vi "move_2.vi"(3 "t":bool, 4 "Array in":i32[](array[numeric]), 5 "Enum 3":enum16{"move2_1", "move2_2"}(ring)) -> (0 "Enum":T1(ring), 1 "Array out":i32[](array[numeric]), 2 "Enum 2":enum16{"move2_1", "move2_2"}(ring))   [LabVIEW 2016]
uses:
  <vilib>/NXT/Block Support/NXT_OutputPort.ctl
  <vilib>/NXT/NXTIO Xnodes/NXTIONodeSubVIs/NXTStopMotors.vi
  <vilib>/NXT/NXTIO Xnodes/NXTIONodeSubVIs/NXTMotorRunDistance.vi
  <vilib>/NXT/NXTIO Xnodes/NXTIONodeSubVIs/LEGOMotorStatus.vi
  <vilib>/NXT/NXTIO Xnodes/NXTIONodeSubVIs/NXTMoveMotors.vi
  <vilib>/NXT/NXTIO Xnodes/NXTIONodeSubVIs/LEGOResetMotors.vi
  <vilib>/NXT/Dual Mode Library/Display/drawText.vi
  <vilib>/NXT/Subs/LVHSConnector.ctl
  <vilib>/NXT/NXTIO Xnodes/AddressXNode/NXTIOAddress.xnode
  <vilib>/NXT/NXTIO Xnodes/NXTIOXNode/NXTIO.xnode
  <vilib>/NXT/LegoClasses/BrickReference/BrickReference.lvclass
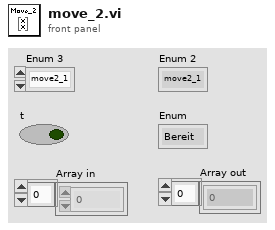
[diagram p1: front panel]
types:
  T1 = enum16{"Bereit", "Move 1", "Reference_pos", "Wait", "row1_check", "row2_check", "row3_check", "return", "move2", "move3", "move4", "move5", "end"}
  T2 = enum16{"forward", "right", "mark", "pause", "up", "return", "end"}
  T3 = typedef "NXT_OutputPort.ctl" = u8
  T4 = cluster{"Output Port":T3, "Output Port 2":T3, "Output Port 3":T3}
  T5 = enum16{"forward", "mark", "pause", "up", "return", "end"}
  T6 = typedef "LVHSConnector.ctl" = refnum<class "BrickReference.lvclass">
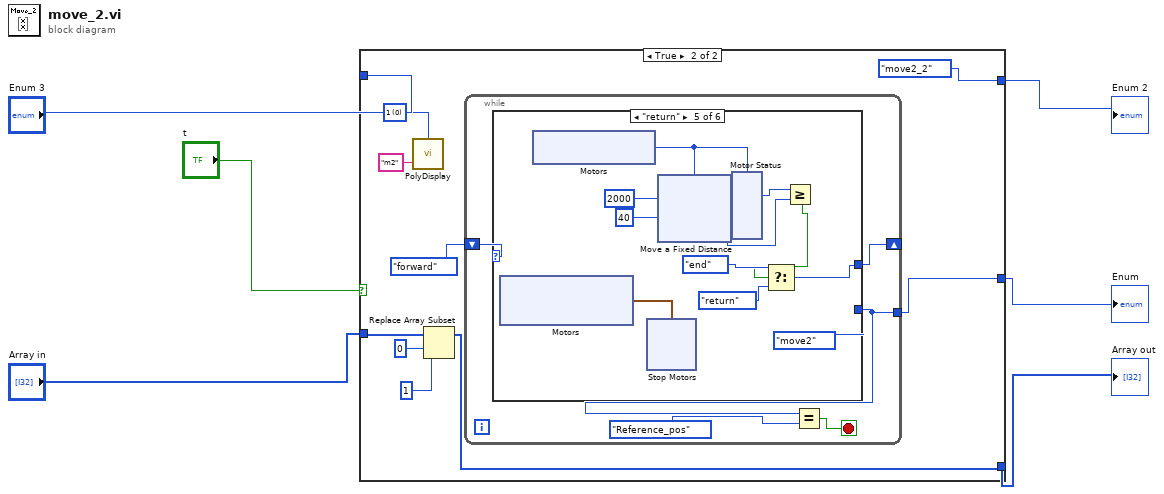
[diagram p0: block diagram]
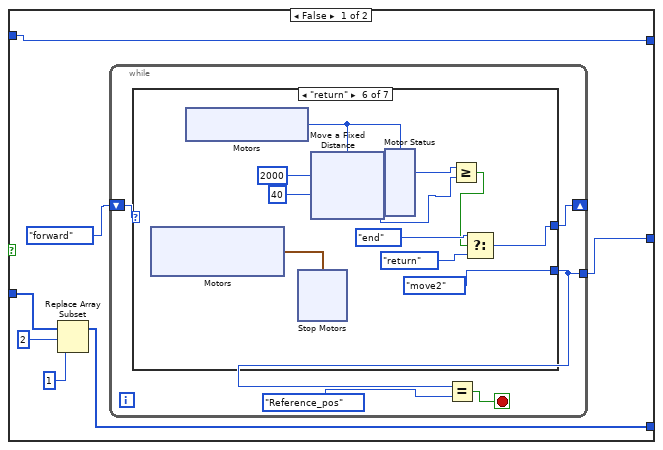
[diagram p2: hidden frame]
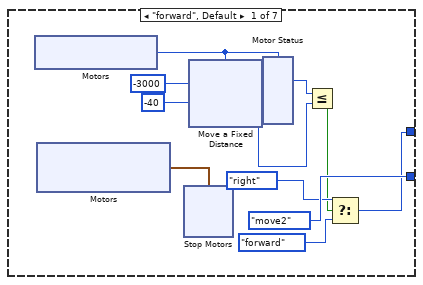
[diagram p3: hidden frame]
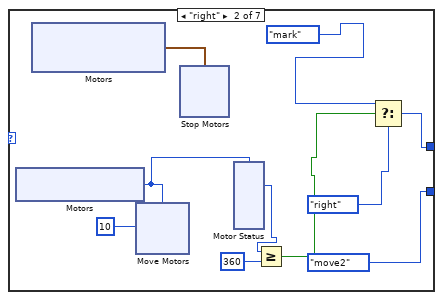
[diagram p4: hidden frame]
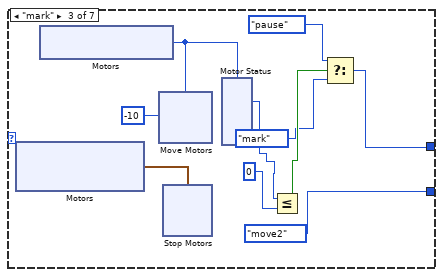
[diagram p5: hidden frame]
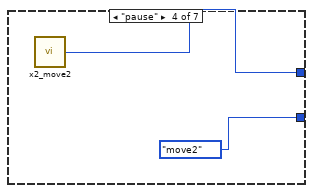
[diagram p6: hidden frame]
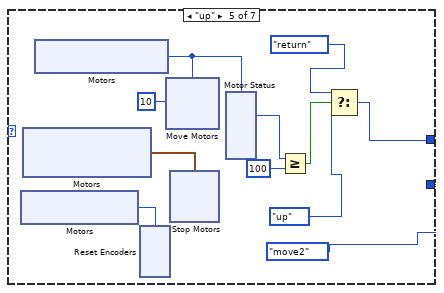
[diagram p7: hidden frame]
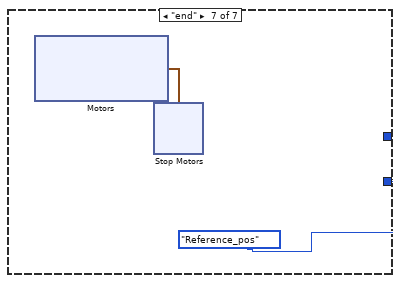
[diagram p8: hidden frame]
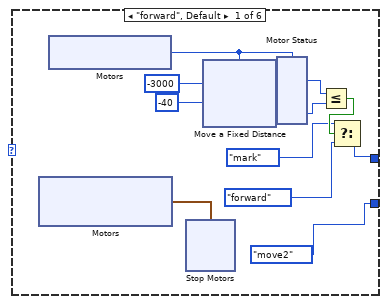
[diagram p9: hidden frame]
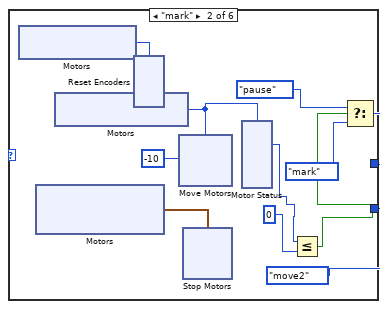
[diagram p10: hidden frame]
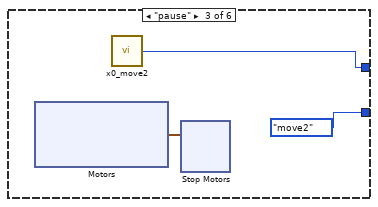
[diagram p11: hidden frame]
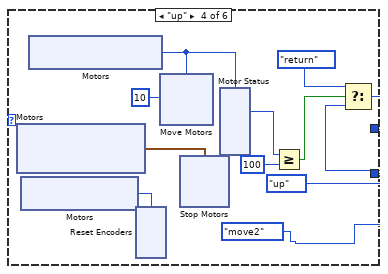
[diagram p12: hidden frame]
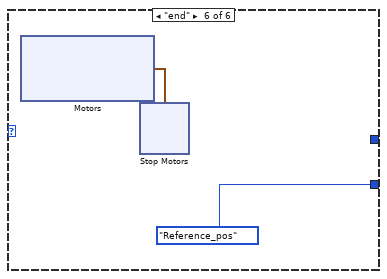
[diagram p13: hidden frame]
diagram:
  n1 = case shown="True" "t" {
    tunnel: [w12 w210] -> w3
    tunnel: "Array in" -> [w9 w207]
    tunnel: [w8 w206] -> w4
    tunnel: "Enum 3" -> [w7 _]
    tunnel: [w7 enum16{"move2_1", "move2_2"}."move2_2"] -> w2
    frame False {
      n2 = Replace Array Subset(array=w9, new element=1 ("new element/subarray"), index=2 ("index (row)")) -> (w8:i32[])
      n3 = while {
        shift-right: [w14] -> _
        shift-left: T2."forward" -> [w15]
        tunnel: [w18] -> w12
        stop <- w17 stop-if-true
        n4 = case shown="\"return\"" w15 {
          tunnel: [w20 w56 w88 w119 w122 w162 _] -> w14
          tunnel: [T1."move2" T1."move2" T1."move2" T1."move2" T1."move2" T1."move2" T1."Reference_pos"] -> w18
          frame "forward", Default {
            w25 = -3000 ("Distance 1")
            n5 = xnode "Motors"() -> ("Motor"=w24:T3)
            n6 = xnode "Motors"() -> ("Motor"=w29:cluster{"Port":T3, "Port":T3})
            n7 = xnode "Stop Motors"("Motors"=w29) -> ()  [unwired: 1 in, 1 out]
            n8 = xnode "Move a Fixed Distance"("Speed 1"=i8 -40, "Distance 1"=w25, "Motors"=w24) -> ("NXT/EV3"=w23:T6)  [unwired: 1 in]
            n9 = xnode "Motor Status"("Motors"=w24, "NXT/EV3"=w23) -> ("Position 1"=w26:i32)  [unwired: 2 out]
            n10 = Less Or Equal?(x=w26, y=w25) -> (x <= y?=w21:bool)
            n11 = Select(t=T2."right", s=w21, f=T2."forward") -> (s? t:f=w20:T2)
          }
          frame "right" {
            n12 = xnode "Motors"() -> ("Motor"=w64:T3)
            n13 = xnode "Motors"() -> ("Motor"=w63:cluster{"Port":T3, "Port":T3})
            n14 = xnode "Move Motors"("Power/Speed 1"=i8 10, "Motors"=w64) -> ()  [unwired: 1 in, 1 out]
            n15 = xnode "Stop Motors"("Motors"=w63) -> ()  [unwired: 1 in, 1 out]
            n16 = xnode "Motor Status"("Motors"=w64) -> ("Position 1"=w61:i32)  [unwired: 1 in, 2 out]
            n17 = Greater Or Equal?(x=w61, y=360) -> (x >= y?=w60:bool)
            n18 = Select(t=T2."mark", s=w60, f=T2."right") -> (s? t:f=w56:T2)
          }
          frame "mark" {
            n19 = xnode "Motors"() -> ("Motor"=w96:cluster{"Port":T3, "Port":T3})
            n20 = xnode "Motors"() -> ("Motor"=w94:T3)
            n21 = xnode "Move Motors"("Power/Speed 1"=i8 -10, "Motors"=w94) -> ()  [unwired: 1 in, 1 out]
            n22 = xnode "Stop Motors"("Motors"=w96) -> ()  [unwired: 1 in, 1 out]
            n23 = xnode "Motor Status"("Motors"=w94) -> ("Position 1"=w93:i32)  [unwired: 1 in, 2 out]
            n24 = Less Or Equal?(x=w93, y=0) -> (x <= y?=w91:bool)
            n25 = Select(t=T2."pause", s=w91, f=T2."mark") -> (s? t:f=w88:T2)
          }
          frame "pause" {
            n26 = call "x2_move2.vi"() -> ("Enum"=w119:T2)  [unwired: 1 in]
          }
          frame "up" {
            n27 = xnode "Motors"() -> ("Motor"=w121:T3)
            n28 = xnode "Motors"() -> ("Motor"=w129:cluster{"Port":T3, "Port":T3})
            n29 = xnode "Motors"() -> ("Motor"=w126:T3)
            n30 = xnode "Reset Encoders"("Motors"=w121) -> ()  [unwired: 1 in, 1 out]
            n31 = xnode "Move Motors"("Power/Speed 1"=i8 10, "Motors"=w126) -> ()  [unwired: 1 in, 1 out]
            n32 = xnode "Stop Motors"("Motors"=w129) -> ()  [unwired: 1 in, 1 out]
            n33 = xnode "Motor Status"("Motors"=w126) -> ("Position 1"=w127:i32)  [unwired: 1 in, 2 out]
            n34 = Greater Or Equal?(x=w127, y=100) -> (x >= y?=w128:bool)
            n35 = Select(t=T2."return", s=w128, f=T2."up") -> (s? t:f=w122:T2)
          }
          frame "return" {
            w160 = 2000 ("Distance 1")
            n36 = xnode "Motors"() -> ("Motor"=w168:cluster{"Port":T3, "Port":T3})
            n37 = xnode "Motors"() -> ("Motor"=w166:T3)
            n38 = xnode "Stop Motors"("Motors"=w168) -> ()  [unwired: 1 in, 1 out]
            n39 = xnode "Move a Fixed Distance"("Speed 1"=i8 40, "Distance 1"=w160, "Motors"=w166) -> ("NXT/EV3"=w165:T6)  [unwired: 1 in]
            n40 = xnode "Motor Status"("Motors"=w166, "NXT/EV3"=w165) -> ("Position 1"=w161:i32)  [unwired: 2 out]
            n41 = Greater Or Equal?(x=w161, y=w160) -> (x >= y?=w159:bool)
            n42 = Select(t=T2."end", s=w159, f=T2."return") -> (s? t:f=w162:T2)
          }
          frame "end" {
            n43 = xnode "Motors"() -> ("Motor"=w195:cluster{"Port":T3, "Port":T3, "Port":T3})
            n44 = xnode "Stop Motors"("Motors"=w195) -> ()  [unwired: 1 in, 1 out]
          }
        }
        n45 = Equal?(x=w18, y=T1."Reference_pos") -> (x = y?=w17:bool)
      }
    }
    frame True {
      w204 = i16 0 items=["1", "2", "3", "4", "5", "6", "7", "8", "9", "10", "11", "12"] ("Line")
      n46 = call-poly <vilib>:"PolyDisplay.vi"("Text"="m2", "Line"=w204) -> ()  [unwired: 2 in, 1 out]
      n47 = Replace Array Subset(array=w207, new element=1 ("new element/subarray"), index=0 ("index (row)")) -> (w206:i32[])
      n48 = while {
        shift-right: [w212] -> _
        shift-left: T5."forward" -> [w216]
        tunnel: [w215] -> w210
        stop <- w214 stop-if-true
        n49 = case shown="\"return\"" w216 {
          tunnel: [w217 w261 w292 w307 w341 _] -> w212
          tunnel: [T1."move2" T1."move2" T1."move2" T1."move2" T1."move2" T1."Reference_pos"] -> w215
          frame "forward", Default {
            w221 = -3000 ("Distance 1")
            n50 = xnode "Motors"() -> ("Motor"=w227:cluster{"Port":T3, "Port":T3})
            n51 = xnode "Motors"() -> ("Motor"=w223:T3)
            n52 = xnode "Stop Motors"("Motors"=w227) -> ()  [unwired: 1 in, 1 out]
            n53 = xnode "Move a Fixed Distance"("Speed 1"=i8 -40, "Distance 1"=w221, "Motors"=w223) -> ("NXT/EV3"=w222:T6)  [unwired: 1 in]
            n54 = xnode "Motor Status"("Motors"=w223, "NXT/EV3"=w222) -> ("Position 1"=w224:i32)  [unwired: 2 out]
            n55 = Less Or Equal?(x=w224, y=w221) -> (x <= y?=w220:bool)
            n56 = Select(t=T5."mark", s=w220, f=T5."forward") -> (s? t:f=w217:T5)
          }
          frame "mark" {
            n57 = xnode "Motors"() -> ("Motor"=w253:T3)
            n58 = xnode "Motors"() -> ("Motor"=w263:cluster{"Port":T3, "Port":T3})
            n59 = xnode "Motors"() -> ("Motor"=w258:T3)
            n60 = xnode "Reset Encoders"("Motors"=w253) -> ()  [unwired: 1 in, 1 out]
            n61 = xnode "Move Motors"("Power/Speed 1"=i8 -10, "Motors"=w258) -> ()  [unwired: 1 in, 1 out]
            n62 = xnode "Stop Motors"("Motors"=w263) -> ()  [unwired: 1 in, 1 out]
            n63 = xnode "Motor Status"("Motors"=w258) -> ("Position 1"=w257:i32)  [unwired: 1 in, 2 out]
            n64 = Less Or Equal?(x=w257, y=0) -> (x <= y?=w255:bool)
            n65 = Select(t=T5."pause", s=w255, f=T5."mark") -> (s? t:f=w261:T5)
          }
          frame "pause" {
            n66 = xnode "Motors"() -> ("Motor"=w291:cluster{"Port":T3, "Port":T3, "Port":T3})
            n67 = call "x0_move2.vi"() -> ("Enum"=w292:T5)  [unwired: 1 in]
            n68 = xnode "Stop Motors"("Motors"=w291) -> ()  [unwired: 1 in, 1 out]
          }
          frame "up" {
            n69 = xnode "Motors"() -> ("Motor"=w309:cluster{"Port":T3, "Port":T3})
            n70 = xnode "Motors"() -> ("Motor"=w300:T3)
            n71 = xnode "Motors"() -> ("Motor"=w303:T3)
            n72 = xnode "Reset Encoders"("Motors"=w300) -> ()  [unwired: 1 in, 1 out]
            n73 = xnode "Move Motors"("Power/Speed 1"=i8 10, "Motors"=w303) -> ()  [unwired: 1 in, 1 out]
            n74 = xnode "Stop Motors"("Motors"=w309) -> ()  [unwired: 1 in, 1 out]
            n75 = xnode "Motor Status"("Motors"=w303) -> ("Position 1"=w304:i32)  [unwired: 1 in, 2 out]
            n76 = Greater Or Equal?(x=w304, y=100) -> (x >= y?=w308:bool)
            n77 = Select(t=T5."return", s=w308, f=T5."up") -> (s? t:f=w307:T5)
          }
          frame "return" {
            w339 = 2000 ("Distance 1")
            n78 = xnode "Motors"() -> ("Motor"=w348:cluster{"Port":T3, "Port":T3})
            n79 = xnode "Motors"() -> ("Motor"=w345:T3)
            n80 = xnode "Stop Motors"("Motors"=w348) -> ()  [unwired: 1 in, 1 out]
            n81 = xnode "Move a Fixed Distance"("Speed 1"=i8 40, "Distance 1"=w339, "Motors"=w345) -> ("NXT/EV3"=w344:T6)  [unwired: 1 in]
            n82 = xnode "Motor Status"("Motors"=w345, "NXT/EV3"=w344) -> ("Position 1"=w340:i32)  [unwired: 2 out]
            n83 = Greater Or Equal?(x=w340, y=w339) -> (x >= y?=w338:bool)
            n84 = Select(t=T5."end", s=w338, f=T5."return") -> (s? t:f=w341:T5)
          }
          frame "end" {
            n85 = xnode "Motors"() -> ("Motor"=w375:cluster{"Port":T3, "Port":T3, "Port":T3})
            n86 = xnode "Stop Motors"("Motors"=w375) -> ()  [unwired: 1 in, 1 out]
          }
        }
        n87 = Equal?(x=w215, y=T1."Reference_pos") -> (x = y?=w214:bool)
      }
    }
  }
  "Array out" <- w4
  "Enum" <- w3
  "Enum 2" <- w2
